vi "GetParam.vi"(11 "添加的路径":path) -> (2 "数组":dbl[](array[numeric]), 3 "路径输出":path caption="路径副本")   [LabVIEW 2018]
uses:
  <vilib>/Utility/file.llb/Write Delimited Spreadsheet (DBL).vi
  <vilib>/Utility/file.llb/Read Delimited Spreadsheet (DBL).vi
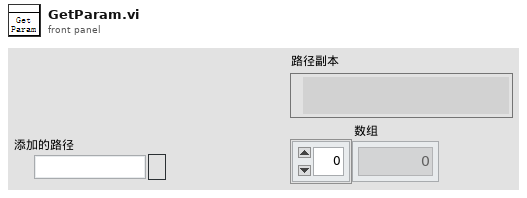
[diagram p1: front panel]
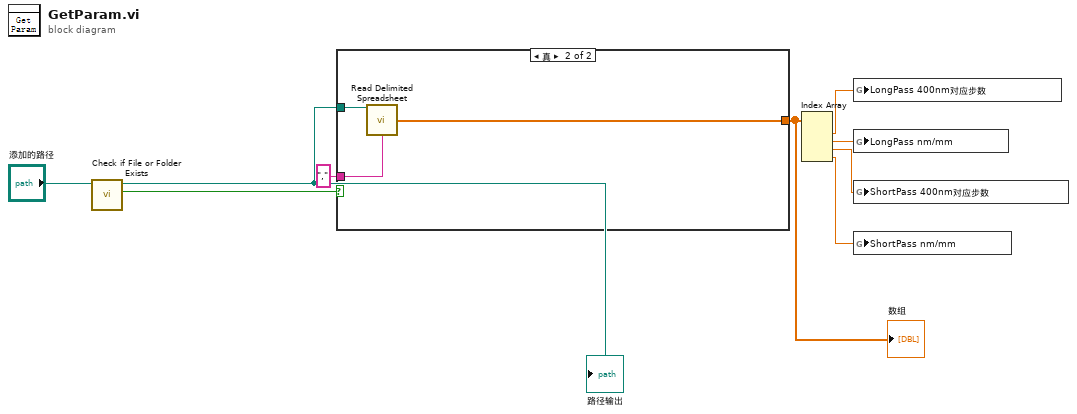
[diagram p0: block diagram]
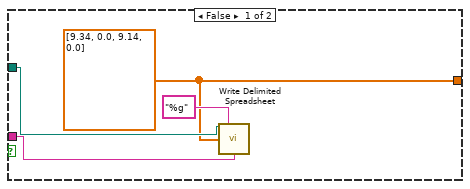
[diagram p2: hidden frame]
diagram:
  n1 = call <vilib>:"Check if File or Folder Exists.vi"("path"="添加的路径") -> ("file or folder exists?"=w8:bool, "dup path"=w7:path)  [unwired: 8 in, 1 out]
  "路径输出" <- w7
  n2 = case shown="真" w8 {
    tunnel: w7 -> [w13 w16]
    tunnel: [w11 w14] -> w1
    tunnel: "," ("delimiter (\\t)") -> [w10 w15]
    frame False {
      w11 = dbl[] [9.34, 0.0, 9.14, 0.0] ("1D data")
      n3 = call-poly <vilib>:"Write Delimited Spreadsheet.vi"("file path (dialog if empty)"=w13, "format (%.3f)"="%g", "1D data"=w11, "delimiter (\\t)"=w10) -> ()  [unwired: 10 in, 2 out]
    }
    frame True {
      n4 = call-poly <vilib>:"Read Delimited Spreadsheet.vi"("file path (dialog if empty)"=w16, "delimiter (\\t)"=w15) -> ("first row"=w14:dbl[])  [unwired: 8 in, 5 out]
    }
  }
  "数组" <- w1
  n5 = Index Array(array=w1) -> (element #1=w4:dbl, element #2=w5:dbl, element #3=w2:dbl, element #4=w3:dbl)  [unwired: 4 in]
  n6 = global write "消息通知.vi" "LongPass 400nm对应步数"(w4) -> ()
  n7 = global write "消息通知.vi" "LongPass nm/mm"(w5) -> ()
  n8 = global write "消息通知.vi" "ShortPass 400nm对应步数"(w2) -> ()
  n9 = global write "消息通知.vi" "ShortPass nm/mm"(w3) -> ()
